vi "Configure Sequence Trigger.vi"(0 "VISA Resource Name":refnum<visa-resource-name>, 1 "edge1 (\"XXXXXXXXXXXXXXXXXX\")":string="XXXXXXXXXXXXXXXXXX" caption="Edge1 (\"XXXXXXXXXXXXXXXXXX\")", 2 "edge number (1)":i32=1 caption="Edge Number (1)", 5 "trigger level (0.0 V)":dbl caption="Trigger Level (0.0 V)" format="%^.2e", 7 "pattern1 (\"XXXXXXXXXXXXXXXXXX\")":string="XXXXXXXXXXXXXXXXXX" caption="Pattern1 (\"XXXXXXXXXXXXXXXXXX\")", 9 "pattern2 (\"XXXXXXXXXXXXXXXXXX\")":string="XXXXXXXXXXXXXXXXXX" caption="Pattern2 (\"XXXXXXXXXXXXXXXXXX\")", 11 "error in (no error)":errorcluster {"code" format="%.0x"}, 12 "edge2 (\"XXXXXXXXXXXXXXXXXX\")":string="XXXXXXXXXXXXXXXXXX" caption="Edge2 (\"XXXXXXXXXXXXXXXXXX\")", 13 "timeout (100.0E-9 sec)":dbl=1e-07 caption="Timeout (100.0E-9 sec)" format="%^.2e") -> (4 "VISA Resource Name Out":refnum<visa-resource-name>, 15 "error out":errorcluster {"code" format="%.0x"})   [LabVIEW 2011, in "Agilent 546XX Series.lvlib"]
doc: "This VI configures the sequence trigger level, pattern (1/2), edge (1/2), number of the edge, and timeout value.\n\nNote: This VI affects instrument behavior only if the trigger type is set to Sequence Trigger. Call the ag546xx Configure Trigger and ag546xx Configure Trigger Coupling VIs to set the trigger type and trigger coupling before calling this VI."
uses:
  Agilent 546XX Series.lvlib
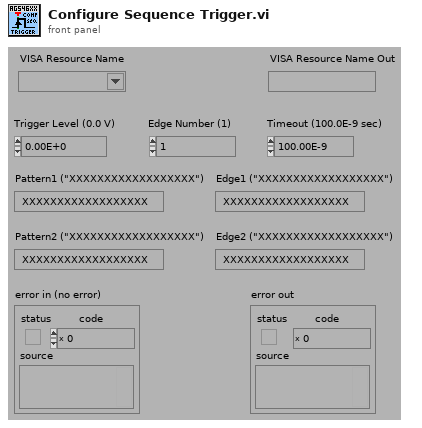
[diagram p1: front panel]
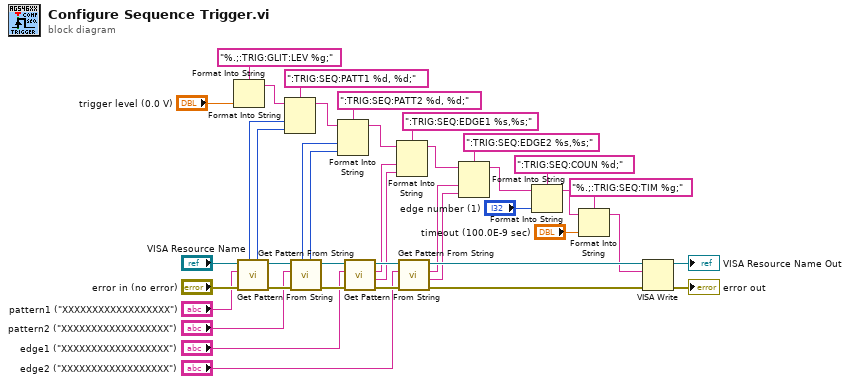
[diagram p0: block diagram]
diagram:
  n1 = Format Into String(format string="%.;:TRIG:GLIT:LEV %g;", "trigger level (0.0 V)") -> (resulting string=w25:string)  [unwired: 2 in, 1 out]
  n2 = call "Get Pattern From String.vi"("error in (no error)"="error in (no error)", "String Pattern (\"XXXXXXXXXXXXXXXXXX\")"="pattern1 (\"XXXXXXXXXXXXXXXXXX\")", "VISA Resource Name"="VISA Resource Name") -> ("error out"=w36:errorcluster, "VISA Resource Name Out"=w37:refnum<visa-resource-name>, "Mask"=w22:u32, "Pattern Value"=w23:u32)  [unwired: 3 in, 2 out]
  n3 = Format Into String(format string=":TRIG:SEQ:PATT1 %d, %d;", initial string=w25, w23, w22) -> (resulting string=w21:string)  [unwired: 1 in, 1 out]
  n4 = call "Get Pattern From String.vi"("error in (no error)"=w36, "String Pattern (\"XXXXXXXXXXXXXXXXXX\")"="pattern2 (\"XXXXXXXXXXXXXXXXXX\")", "VISA Resource Name"=w37) -> ("error out"=w34:errorcluster, "VISA Resource Name Out"=w35:refnum<visa-resource-name>, "Mask"=w19:u32, "Pattern Value"=w20:u32)  [unwired: 3 in, 2 out]
  n5 = Format Into String(format string=":TRIG:SEQ:PATT2 %d, %d;", initial string=w21, w20, w19) -> (resulting string=w16:string)  [unwired: 1 in, 1 out]
  n6 = call "Get Pattern From String.vi"("error in (no error)"=w34, "String Pattern (\"XXXXXXXXXXXXXXXXXX\")"="edge1 (\"XXXXXXXXXXXXXXXXXX\")", "VISA Resource Name"=w35) -> ("error out"=w32:errorcluster, "Slope"=w14:string, "Edge Source"=w15:string, "VISA Resource Name Out"=w33:refnum<visa-resource-name>)  [unwired: 3 in, 2 out]
  n7 = Format Into String(format string=":TRIG:SEQ:EDGE1 %s,%s;", initial string=w16, w15, w14) -> (resulting string=w13:string)  [unwired: 1 in, 1 out]
  n8 = call "Get Pattern From String.vi"("error in (no error)"=w32, "String Pattern (\"XXXXXXXXXXXXXXXXXX\")"="edge2 (\"XXXXXXXXXXXXXXXXXX\")", "VISA Resource Name"=w33) -> ("error out"=w30:errorcluster, "Slope"=w10:string, "Edge Source"=w11:string, "VISA Resource Name Out"=w31:refnum<visa-resource-name>)  [unwired: 3 in, 2 out]
  n9 = Format Into String(format string=":TRIG:SEQ:EDGE2 %s,%s;", initial string=w13, w11, w10) -> (resulting string=w9:string)  [unwired: 1 in, 1 out]
  n10 = Format Into String(format string=":TRIG:SEQ:COUN %d;", initial string=w9, "edge number (1)") -> (resulting string=w5:string)  [unwired: 1 in, 1 out]
  n11 = Format Into String(format string="%.;:TRIG:SEQ:TIM %g;", initial string=w5, "timeout (100.0E-9 sec)") -> (resulting string=w3:string)  [unwired: 1 in, 1 out]
  n12 = VISA Write(VISA resource name=w31, write buffer=w3, error in (no error)=w30) -> (VISA resource name out=→"VISA Resource Name Out":refnum<visa-resource-name>, error out=→"error out":errorcluster)  [unwired: 1 out]
